vi "Process_DoNotRun.vi"(8 "error in":errorcluster, 11 "Logger":refnum<class "Logger.lvclass">) -> (0 "error out":errorcluster, 3 "Logger out":refnum<class "Logger.lvclass">)   [LabVIEW 2019, in "Logger.lvclass"]
doc: "---------------------------------------------------------------\nJKI State Machine Objects™\nhttp://jki.net/state-machine-objects/\nCopyright (C) 2005-2015, JKI <info@jki.net>\nALL RIGHTS RESERVED"
uses:
  Logger.lvclass
  <vilib>/JKI/JKI SMO/SMO/SMO.lvclass
  C:/Program Files (x86)/National Instruments/LabVIEW 2019/vi.lib/JKI/JKI SMO/SMO/SMO.lvclass
panel:
  out "String":string
  # "For instructions on how to use the JKI State Machine Objects, examples and video tutorials, visit:\nhttp://jki.net/state-machine-objects/\n\nJKI State Machine Objects™\nhttp://jki.net/state-machine-objects/\nCopyright (C) 2005-2015, JKI <info@jki.net>\nALL RIGHTS RESERVED"
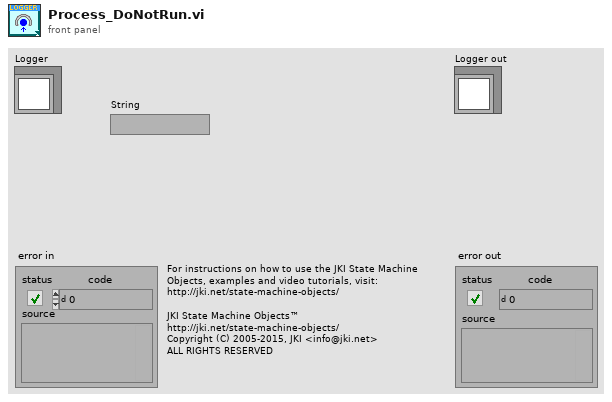
[diagram p1: front panel]
types:
  T1 = enum32{"invalid app kind", "Development System", "Run Time System", "Student Edition", "Embedded LabVIEW", "Evaluation", "Custom"}
  T2 = enum32{"Invalid", "Standard", "Closed", "Hidden", "Minimized", "Maximized"}
  T3 = enum32{"Bad", "Idle", "Run top level", "Running"}
  T4 = cluster{"Core":cluster{"Current VI Reference":refnum<vi>, "Close Panel on Exit?":bool, "error":errorcluster}, "Self Reference":refnum<class "Logger.lvclass">, "Debug Mode?":bool}
  T5 = cluster{"Current VI Reference":refnum<vi>, "Close Panel on Exit?":bool, "error":errorcluster}
  T6 = typedef "SMO.lvclass/Protected Events.ctl" = cluster{"StopProcesses":refnum<user-event>, "AbortProcesses":refnum<user-event>, "Config Changed":refnum<user-event>, "Dependency":refnum<user-event>}
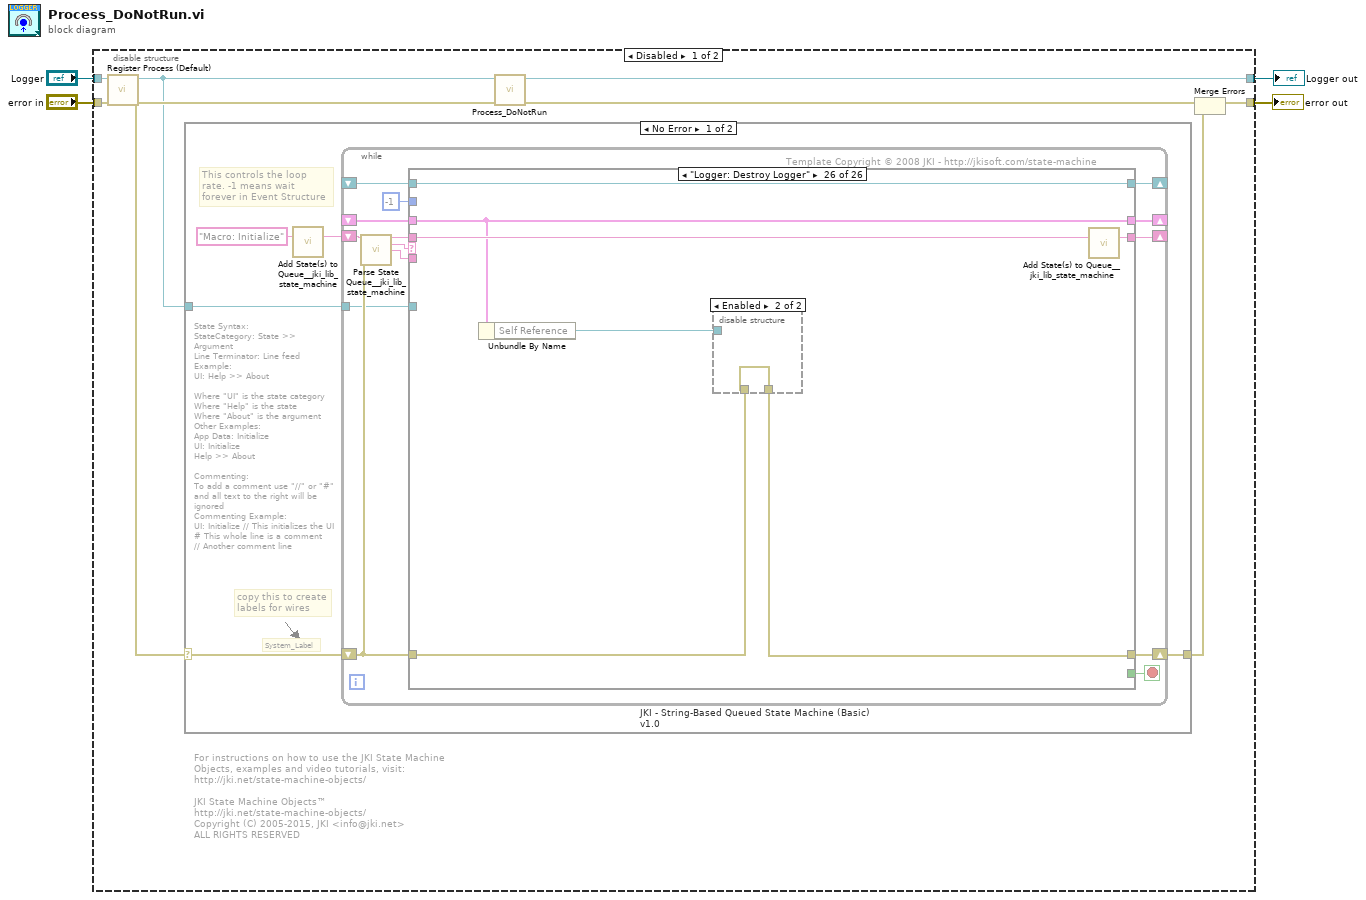
[diagram p0: block diagram]
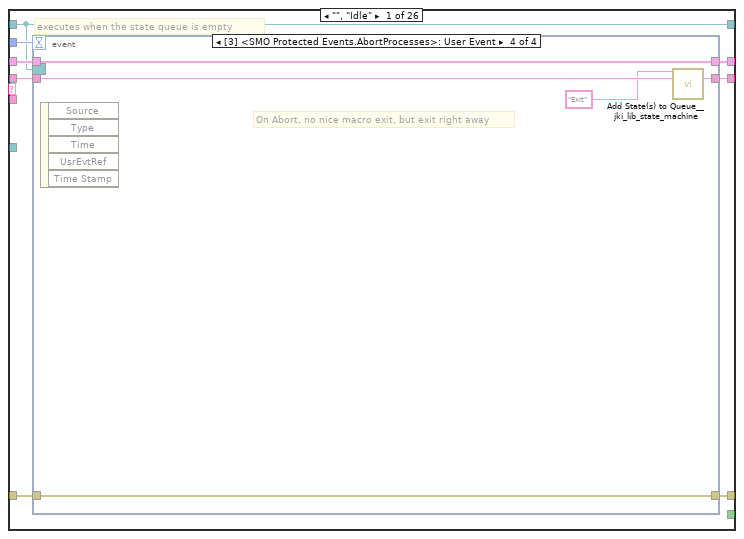
[diagram p2: hidden frame]
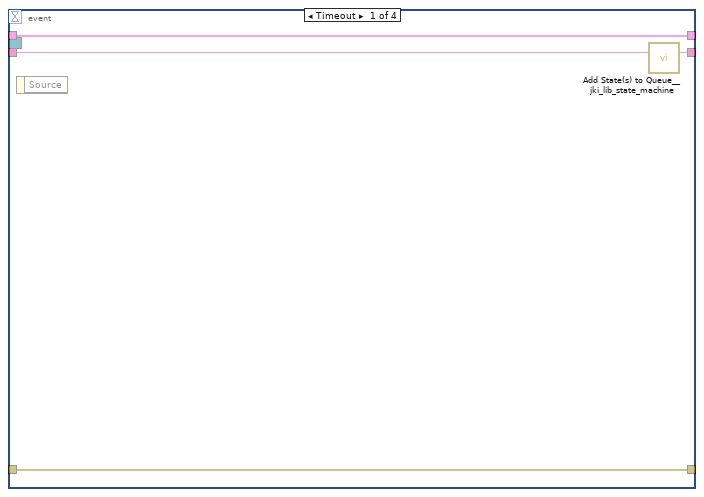
[diagram p3: hidden frame]
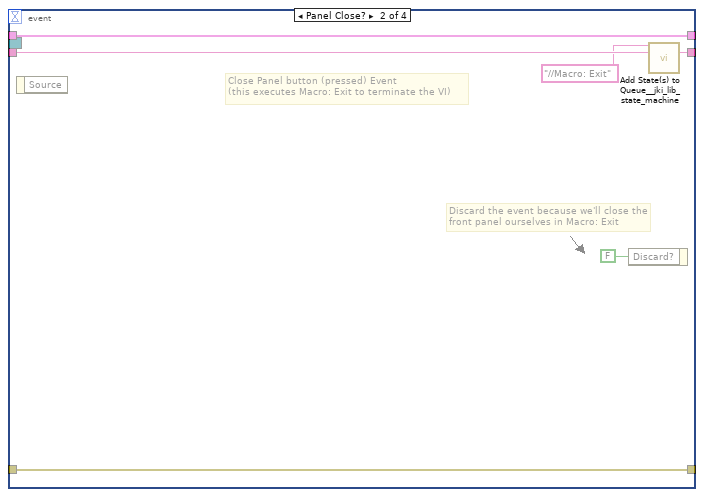
[diagram p4: hidden frame]
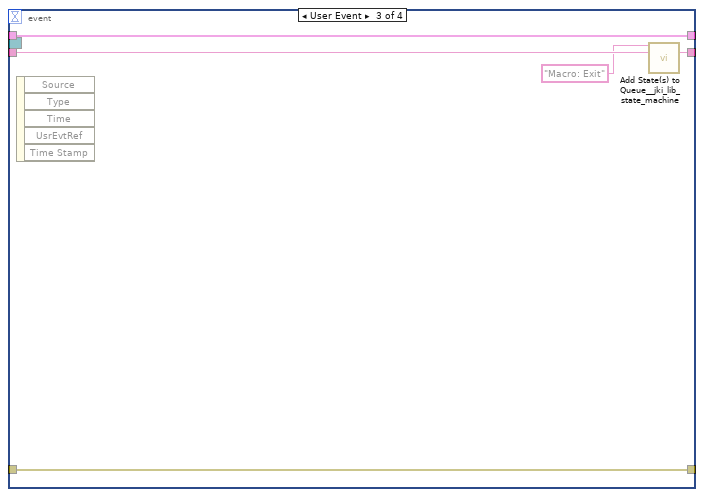
[diagram p5: hidden frame]
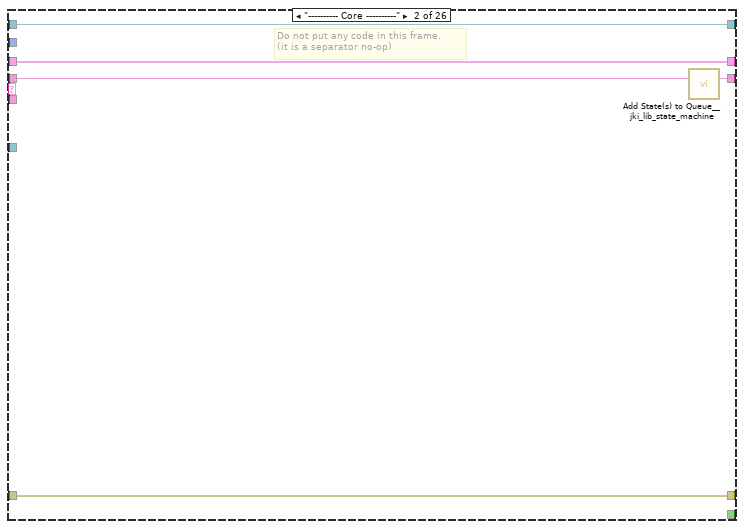
[diagram p6: hidden frame]
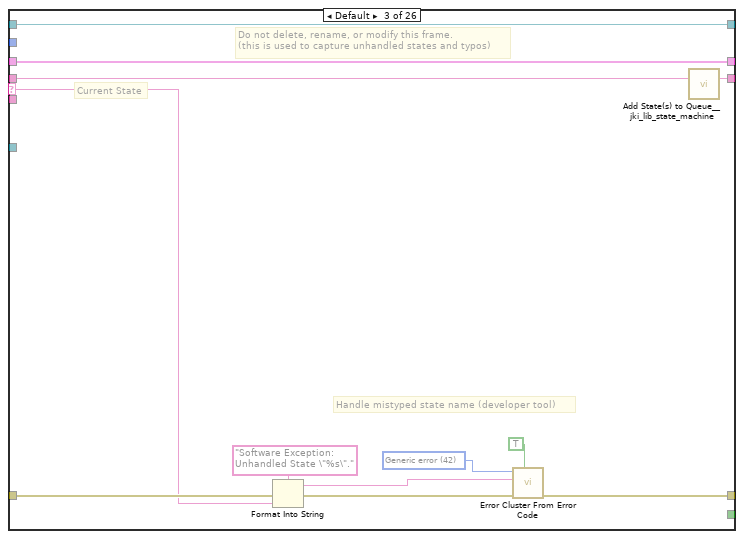
[diagram p7: hidden frame]
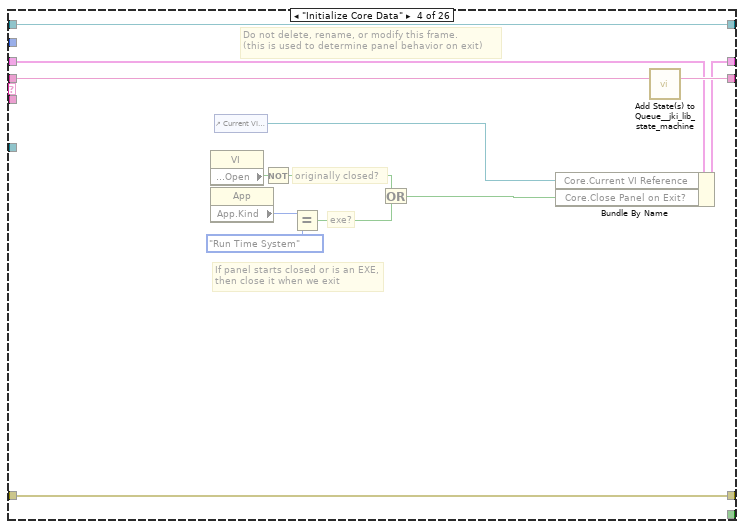
[diagram p8: hidden frame]
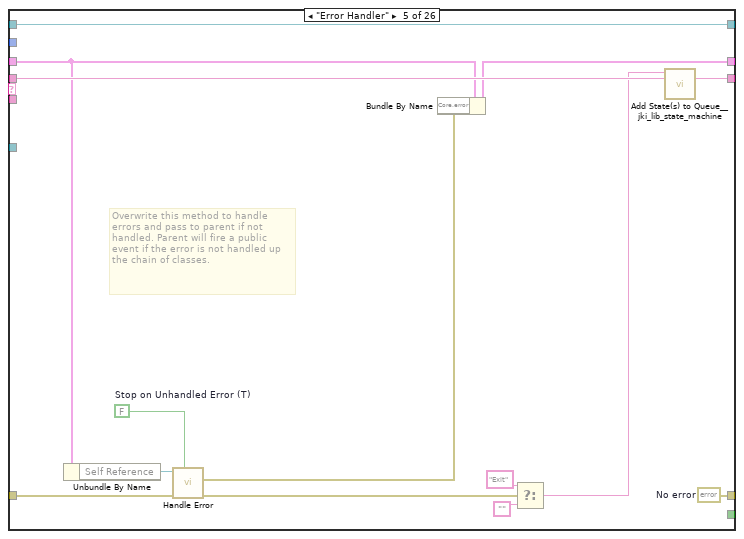
[diagram p9: hidden frame]
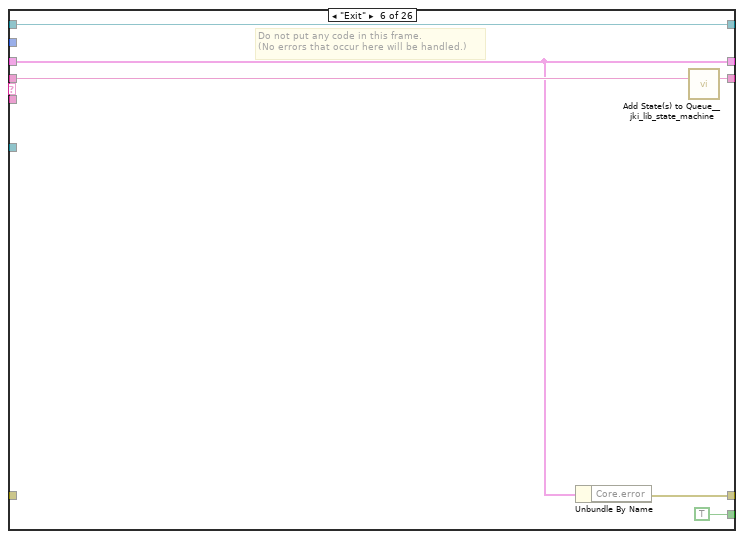
[diagram p10: hidden frame]
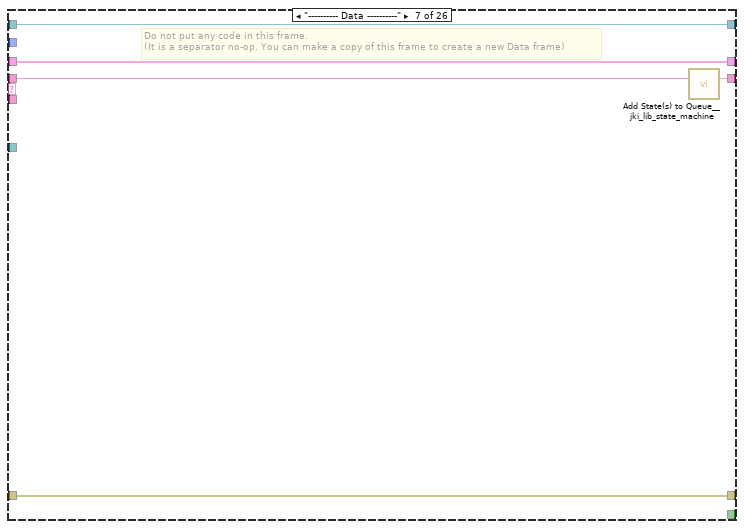
[diagram p11: hidden frame]
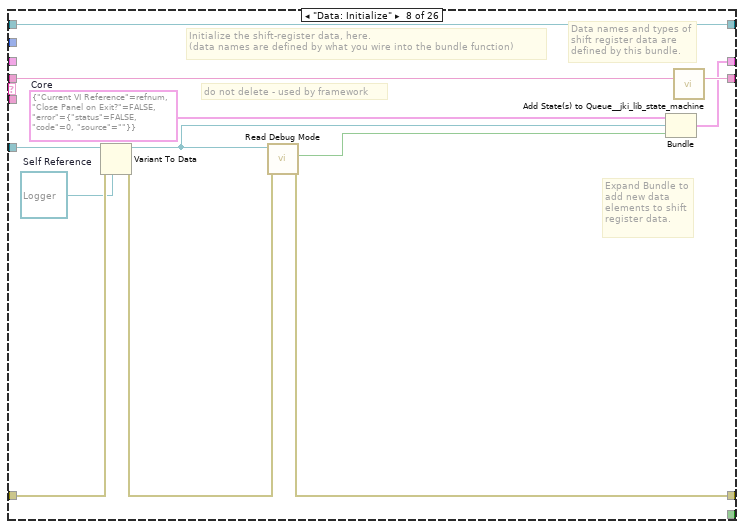
[diagram p12: hidden frame]
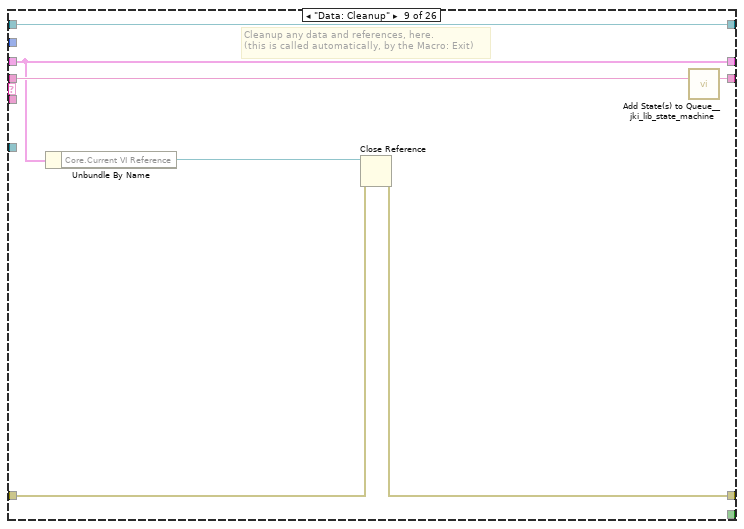
[diagram p13: hidden frame]
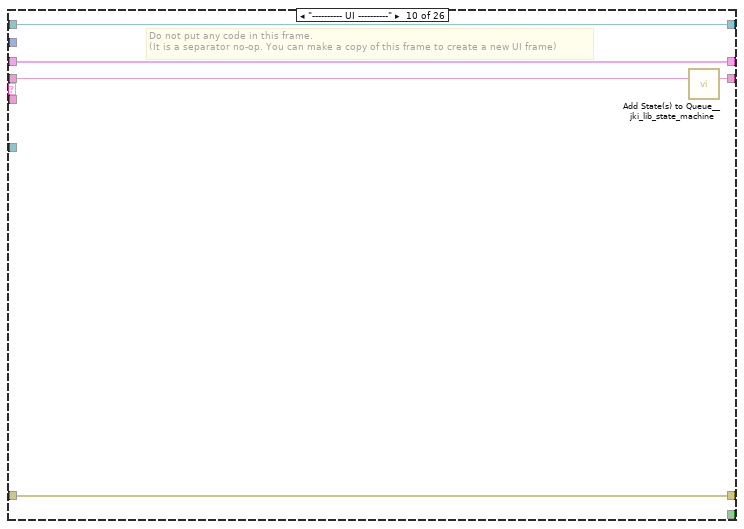
[diagram p14: hidden frame]
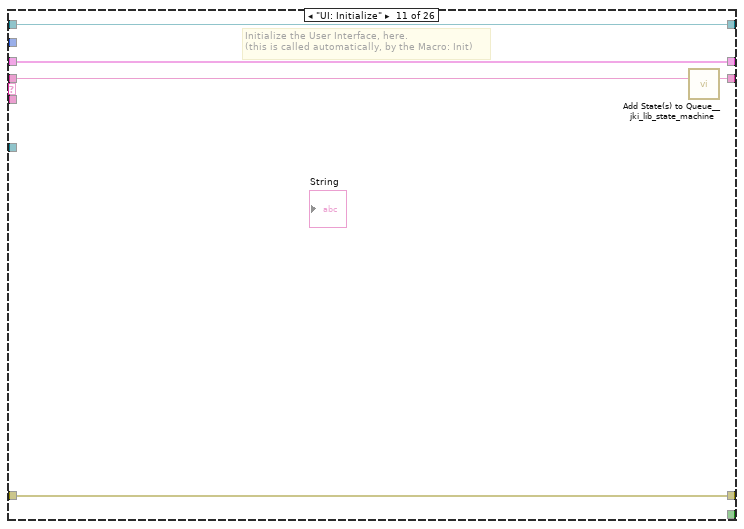
[diagram p15: hidden frame]
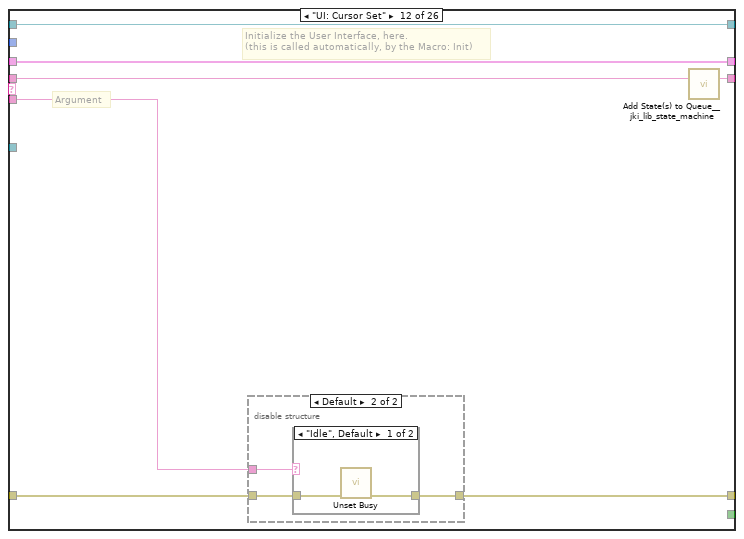
[diagram p16: hidden frame]
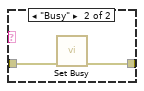
[diagram p18: hidden frame]
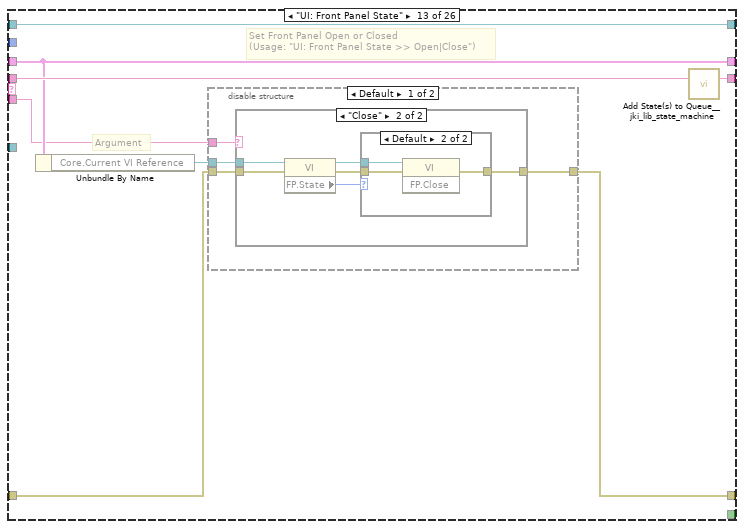
[diagram p19: hidden frame]
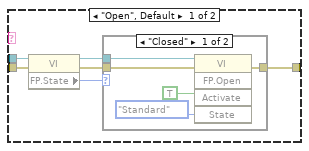
[diagram p20: hidden frame]
diagram:
  n1 = disable-structure shown="Disabled" {
    disable-tunnel: "Logger" -> [w12 w321]
    disable-tunnel: "error in" -> [w11 w320]
    disable-tunnel: [w10 w320] -> w2
    disable-tunnel: [w7 w321] -> w1
    frame Disabled {
      # "For instructions on how to use the JKI State Machine Objects, examples and video tutorials, visit:\nhttp://jki.net/state-machine-objects/\n\nJKI State Machine Objects™\nhttp://jki.net/state-machine-objects/\nCopyright (C) 2005-2015, JKI <info@jki.net>\nALL RIGHTS RESERVED"
      n2 = call <vilib>:"Register Process (Default).vi"("error in (no error)"=w11, "SMO"=w12) -> ("error out"=w9:errorcluster, "SelfRef"=w8:refnum<class "Logger.lvclass">)  [unwired: 8 in]
      n3 = case shown="No Error" w9 {
        selector: w9 -> [w14 w319]
        tunnel: w8 -> [w15 _]
        tunnel: [w13 w319] -> w5
        frame No Error {
          # "State Syntax:\nStateCategory: State >> Argument\nLine Terminator: Line feed\nExample:\nUI: Help >> About\n\nWhere \"UI\" is the state category\nWhere \"Help\" is the state\nWhere \"About\" is the argument\nOther Examples:\nApp Data: Initialize\nUI: Initialize\nHelp >> About\n\nCommenting:\nTo add a comment use \"//\" or \"#\" and all text to the right will be ignored\nCommenting Example:\nUI: Initialize // This initializes the UI\n# This whole line is a comment\n// Another comment line"
          # "copy this to create labels for wires"
          # "This controls the loop rate. -1 means wait forever in Event Structure"
          # "System_Label"
          n4 = call <vilib>:"Add State(s) to Queue__jki_lib_state_machine.vi"("State(s) in (\"\")"="Macro: Initialize") -> ("States Out"=w17:string)  [unwired: 14 in]
          n5 = while "JKI - String-Based Queued State Machine (Basic) v1.0" {
            shift-right: [w24] -> _
            shift-left: _ -> [w23]
            shift-right: [w27] -> w13
            shift-left: w14 -> [w21]
            shift-right: [w26] -> _
            shift-left: w17 -> [w28]
            tunnel: w15 -> [w20]
            shift-right: [w19] -> _
            shift-left: _ -> [w18]
            stop <- w25 stop-if-true
            # "Template Copyright © 2008 JKI - http://jkisoft.com/state-machine"
            n6 = call <vilib>:"Parse State Queue__jki_lib_state_machine.vi"("State Queue"=w28, "Error In (no error)"=w21) -> ("Remaining States"=w30:string, "Current State"=w31:string, "Arguments"=w29:string)  [unwired: 11 in]
            n7 = case shown="\"Logger: Destroy Logger\"" w31 {
              selector: w31 -> [_ _ w66 _ _ _ _ _ _ _ _ _ _ _ _ _ _ _ _ _ _ _ _ _ _ _]
              tunnel: w30 -> [w39 w64 w70 w89 w103 w109 w114 w126 w133 w138 w143 w150 w166 w198 w221 w240 w245 w256 w261 w271 w277 w282 w291 w302 w307 w314]
              tunnel: w29 -> [_ _ _ _ _ _ _ _ _ _ _ w144 w160 _ _ _ _ _ _ _ _ _ _ _ _ _]
              tunnel: w23 -> [w37 w61 w68 w80 w97 w105 w111 _ w128 w135 w141 w148 w162 w195 w203 w232 w242 w246 w258 w269 w275 w280 w288 w298 w303 w311]
              tunnel: [w36 w62 w72 w86 w98 w104 w112 w115 w129 w136 w140 w145 w163 w196 w199 w238 w243 w248 w259 w264 w273 w278 w283 w299 w304 w308] -> w27
              tunnel: w21 -> [w35 w62 w71 w86 w99 _ w112 w123 w130 w136 w140 w146 w164 w196 w200 w238 w243 w249 w259 w265 w273 w278 w284 w299 w304 w309]
              tunnel: [w38 w63 w69 w88 w102 w108 w113 w125 w132 w137 w142 w149 w165 w197 w220 w239 w244 w255 w260 w270 w276 w281 w290 w301 w306 w313] -> w26
              tunnel: [_ _ _ _ _ TRUE _ _ _ _ _ _ _ _ _ _ _ _ _ _ _ _ _ _ _ _] -> w25
              tunnel: [w34 w61 w68 w87 w96 w105 w111 w124 w128 w135 w141 w148 w162 w195 w203 w232 w242 w246 w258 w269 w275 w280 w287 w298 w303 w311] -> w24
              tunnel: -1 ("Timeout") -> [w33 _ _ _ _ _ _ _ _ _ _ _ _ _ _ _ _ _ _ _ _ _ _ _ _ _]
              tunnel: w20 -> [_ _ _ _ _ _ _ w121 _ _ _ _ _ _ w201 _ _ _ _ _ _ _ _ _ _ _]
              tunnel: [w32 w60 w65 w77 w101 w106 w110 w120 w127 w134 w139 w147 w159 w194 w219 w233 w241 w254 w257 w268 w274 w279 w289 w300 w305 w312] -> w19
              tunnel: w18 -> [w32 w60 w65 w77 w101 w106 w110 w120 w127 w134 w139 w147 w159 w194 w219 w233 w241 w254 w257 _ w274 w279 w289 w300 w305 w312]
              frame "", "Idle" {
                # "executes when the state queue is empty"
                n8 = event shown="[3] <SMO Protected Events.AbortProcesses>: User Event" {
                  selector: w32 -> [_ _ _ _]
                  dyn-events: _ -> [_ _ _ _]
                  timeout: w33 -> [_ _ _ _]
                  tunnel: w39 -> [w43 w49 w54 w59]
                  tunnel: [w42 w48 w53 w58] -> w38
                  tunnel: w37 -> [w41 w46 w51 w56]
                  tunnel: [w40 w47 w52 w57] -> w36
                  tunnel: w35 -> [w40 w47 w52 w57]
                  tunnel: [w41 w46 w51 w56] -> w34
                  event Timeout {
                    n9 = event-data() -> ()  [unwired: 1 in, 1 out]
                    n10 = call <vilib>:"Add State(s) to Queue__jki_lib_state_machine.vi"("State(s) in (\"\")"=w43) -> ("States Out"=w42:string)  [unwired: 14 in]
                  }
                  event Panel Close? {
                    # "Discard the event because we'll close the front panel ourselves in Macro: Exit"
                    # "Close Panel button (pressed) Event\n(this executes Macro: Exit to terminate the VI)"
                    n11 = event-data() -> ()  [unwired: 1 in, 1 out]
                    n12 = event-data("Discard?"=FALSE) -> ()  [unwired: 1 in, 1 out]
                    n13 = call <vilib>:"Add State(s) to Queue__jki_lib_state_machine.vi"("State(s) in Front (\"\")"="//Macro: Exit", "State(s) in (\"\")"=w49) -> ("States Out"=w48:string)  [unwired: 13 in]
                  }
                  event User Event {
                    n14 = event-data() -> ()  [unwired: 1 in, 5 out]
                    n15 = call <vilib>:"Add State(s) to Queue__jki_lib_state_machine.vi"("State(s) in Front (\"\")"="Macro: Exit", "State(s) in (\"\")"=w54) -> ("States Out"=w53:string)  [unwired: 13 in]
                  }
                  event User Event {
                    # "On Abort, no nice macro exit, but exit right away"
                    n16 = event-data() -> ()  [unwired: 1 in, 5 out]
                    n17 = call <vilib>:"Add State(s) to Queue__jki_lib_state_machine.vi"("State(s) in Front (\"\")"="Exit", "State(s) in (\"\")"=w59) -> ("States Out"=w58:string)  [unwired: 13 in]
                  }
                }
              }
              frame "---------- Core ----------" {
                # "Do not put any code in this frame.\n(it is a separator no-op)"
                n18 = call <vilib>:"Add State(s) to Queue__jki_lib_state_machine.vi"("State(s) in (\"\")"=w64) -> ("States Out"=w63:string)  [unwired: 14 in]
              }
              frame Default {
                w75 = 42 items=["No error", "Argument error", "Memory is full", "Out of zone", "End of file", "File already open", "Generic file I/O error", "File not found", "File permission error", "Disk is full", "Duplicate path", "Too many files open", "System feature not enabled", "Resource file not found", "Cannot add resource", "Resource not found", "Image not found", "Image memory error", "Pen does not exist", "Config type invalid", "Config token not found", "Config parse error", "Config memory error", "Bad external code format", "Bad external code offset", "External code not present", "Null window", "Destroy window error", "Null menu", "Print aborted", "Bad print record", "Print driver error", "Windows error during printing", "Memory error during printing", "Print dialog error", "Generic print error", "Invalid device refnum", "Device not found", "Device parameter error", "Device unit error", "Cannot open device", "Device call aborted", "Generic error", "Cancelled by user", "Object ID too low", "Object ID too high", "Object not in heap", "Unknown heap", "Unknown object (invalid DefProc)", "Unknown object (DefProc not in table)", "Message out of range", "Invalid (null) method", "Unknown message", "Manager call not supported", "Bad address", "Network operation in progress", "Network operation timed out", "Connection is busy", "Network attribute not supported", "Network error", "Address in use", "System out of memory", "Connection aborted", "Connection refused", "Not connected", "Already connected", "Connection closed", "Initialization error (interapplication manager)", "Bad occurrence", "Wait on unbound occurrence handler", "Occurrence queue overflow", "Datalog type conflict", "Unused", "Unrecognized type (interapplication manager)", "Memory corrupt", "Failed to make temporary DLL", "Old CIN version", "Drag socket not found", "Failed to load drop-object", "Failed to register OLE object", "Failed to release OLE object", "Format specifier type mismatch", "Unknown format specifier", "Too few format specifiers", "Too many format specifiers", "Scan failed", "Newer CIN version", "Error converting to variant", "Runtime menu error", "Password tampered", "Variant attribute not found", "Incompatible variant data type", "Event data is not available", "Event Store is not present", "Occurrence is not found", "Event Queue is not created", "Event info is not available", "Refnum passed is NULL", "Error retrieving Class GUID", "Error retrieving CoClass GUID", "Error retrieving TypeLib GUID.", "Bad built application magic bytes.", "Specific driver is different from the specific driver associated with the Logical Name.", "There is no session opened to the class driver.", "Max Error", "MAX - Error with config objects", "MAX - Error loading configuration", "MAX - Group not supported"]
                # "Current State"
                # "Do not delete, rename, or modify this frame.\n(this is used to capture unhandled states and typos)"
                # "Handle mistyped state name (developer tool)"
                n19 = Format Into String(format string="Software Exception: Unhandled State \"%s\"." ("message"), error in=w71, w66) -> (resulting string=w74:string, error out=w73:errorcluster)  [unwired: 1 in]
                n20 = call <vilib>:"Error Cluster From Error Code.vi"("show call chain? (False)"=TRUE, "error in (no error)"=w73, "error message (\"\")"=w74, "error code (0)"=w75) -> ("error out"=w72:errorcluster)  [unwired: 5 in]
                n21 = call <vilib>:"Add State(s) to Queue__jki_lib_state_machine.vi"("State(s) in (\"\")"=w70) -> ("States Out"=w69:string)  [unwired: 14 in]
              }
              frame "Initialize Core Data" {
                # "Do not delete, rename, or modify this frame.\n(this is used to determine panel behavior on exit)"
                # "originally closed?"
                # "exe?"
                # "If panel starts closed or is an EXE, then close it when we exit"
                n22 = property class="VI"() -> ("Front Panel.Open"=w85:bool)  [unwired: 2 in, 2 out]
                n23 = property class="App"() -> ("App.Kind"=w84:T1)  [unwired: 2 in, 2 out]
                n24 = control-ref of="Current VI Reference"() -> (w78:refnum<vi>)
                n25 = Not(x=w85) -> (.not. x?=w82:bool)
                n26 = Equal?(x=w84, y=T1."Run Time System" ("Application:Kind")) -> (x = y?=w81:bool)
                n27 = Or(x=w82, y=w81) -> (x .or. y?=w79:bool)
                n28 = Bundle By Name(cluster=w80, "Core.Current VI Reference"=w78, "Core.Close Panel on Exit?"=w79) -> (w87:T4)
                n29 = call <vilib>:"Add State(s) to Queue__jki_lib_state_machine.vi"("State(s) in (\"\")"=w89) -> ("States Out"=w88:string)  [unwired: 14 in]
              }
              frame "Error Handler" {
                w90 = FALSE  # Stop on Unhandled Error (T)
                w98 = errorcluster {"status"=FALSE, "code"=0, "source"=""}  # No error
                # "Overwrite this method to handle errors and pass to parent if not handled. Parent will fire a public event if the error is not handled up the chain of classes."
                n30 = Unbundle By Name(w97) -> ("Self Reference"=w100:refnum<class "Logger.lvclass">)
                n31 = call-dynamic "Handle Error.vi"("Stop on Unhandled Error (T)"=w90, "error in"=w99, "SMO"=w100) -> ("handling error"=w91:errorcluster, "Unhandled error"=w94:errorcluster)  [unwired: 6 in, 1 out]
                n32 = Bundle By Name(cluster=w97, "Core.error"=w94) -> (w96:T4)
                n33 = Select(t="Exit", s=w91, f="") -> (s? t:f=w95:string)
                n34 = call <vilib>:"Add State(s) to Queue__jki_lib_state_machine.vi"("State(s) in Front (\"\")"=w95, "State(s) in (\"\")"=w103) -> ("States Out"=w102:string)  [unwired: 13 in]
              }
              frame "Exit" {
                # "Do not put any code in this frame.\n(No errors that occur here will be handled.)"
                n35 = Unbundle By Name(w105) -> ("Core.error"=w104:errorcluster)
                n36 = call <vilib>:"Add State(s) to Queue__jki_lib_state_machine.vi"("State(s) in (\"\")"=w109) -> ("States Out"=w108:string)  [unwired: 14 in]
              }
              frame "---------- Data ----------" {
                # "Do not put any code in this frame.\n(It is a separator no-op. You can make a copy of this frame to create a new Data frame)"
                n37 = call <vilib>:"Add State(s) to Queue__jki_lib_state_machine.vi"("State(s) in (\"\")"=w114) -> ("States Out"=w113:string)  [unwired: 14 in]
              }
              frame "Data: Initialize" {
                w119 = T5 {"Current VI Reference"=refnum, "Close Panel on Exit?"=FALSE, "error"={"status"=FALSE, "code"=0, "source"=""}}  # Core
                w122 = refnum<class "Logger.lvclass"> refnum  # Self Reference
                # "do not delete - used by framework"
                # "Expand Bundle to add new data elements to shift register data."
                # "Data names and types of shift register data are defined by this bundle."
                # "Initialize the shift-register data, here.\n(data names are defined by what you wire into the bundle function)"
                n38 = Variant To Data(error in=w123, type=w122, Variant=w121) -> (data=w118:refnum<class "Logger.lvclass">, error out=w116:errorcluster)
                n39 = call "Read Debug Mode.vi"("error in (no error)"=w116, "Logger in"=w118) -> ("error out"=w115:errorcluster, "Debug Mode?"=w117:bool)  [unwired: 7 in, 1 out]
                n40 = Bundle("Core"=w119, "Self Reference"=w118, "Debug Mode?"=w117) -> (w124:T4)  [unwired: 1 in]
                n41 = call <vilib>:"Add State(s) to Queue__jki_lib_state_machine.vi"("State(s) in (\"\")"=w126) -> ("States Out"=w125:string)  [unwired: 14 in]
              }
              frame "Data: Cleanup" {
                # "Cleanup any data and references, here.\n(this is called automatically, by the Macro: Exit)"
                n42 = Unbundle By Name(w128) -> ("Core.Current VI Reference"=w131:refnum<vi>)
                n43 = Close Reference(reference=w131, error in (no error)=w130) -> (error out=w129:errorcluster)
                n44 = call <vilib>:"Add State(s) to Queue__jki_lib_state_machine.vi"("State(s) in (\"\")"=w133) -> ("States Out"=w132:string)  [unwired: 14 in]
              }
              frame "---------- UI ----------" {
                # "Do not put any code in this frame.\n(It is a separator no-op. You can make a copy of this frame to create a new UI frame)"
                n45 = call <vilib>:"Add State(s) to Queue__jki_lib_state_machine.vi"("State(s) in (\"\")"=w138) -> ("States Out"=w137:string)  [unwired: 14 in]
              }
              frame "UI: Initialize" {
                # "Initialize the User Interface, here.\n(this is called automatically, by the Macro: Init)"
                n46 = call <vilib>:"Add State(s) to Queue__jki_lib_state_machine.vi"("State(s) in (\"\")"=w143) -> ("States Out"=w142:string)  [unwired: 14 in]
              }
              frame "UI: Cursor Set" {
                # "Argument"
                # "Initialize the User Interface, here.\n(this is called automatically, by the Macro: Init)"
                n47 = disable-structure shown="Default" {
                  disable-tunnel: w146 -> [w151 w154]
                  disable-tunnel: [w151 w153] -> w145
                  disable-tunnel: w144 -> [_ w152]
                  frame condition #0 {
                  }
                  frame condition #1 (active) {
                    n48 = case shown="\"Idle\", Default" w152 {
                      tunnel: w154 -> [w156 w158]
                      tunnel: [w155 w157] -> w153
                      frame "Idle", Default {
                        n49 = call <vilib>:"Unset Busy.vi"("error in (no error)"=w156) -> ("error out"=w155:errorcluster)  [unwired: 10 in]
                      }
                      frame "Busy" {
                        n50 = call <vilib>:"Set Busy.vi"("error in (no error)"=w158) -> ("error out"=w157:errorcluster)  [unwired: 9 in, 1 out]
                      }
                    }
                  }
                }
                n51 = call <vilib>:"Add State(s) to Queue__jki_lib_state_machine.vi"("State(s) in (\"\")"=w150) -> ("States Out"=w149:string)  [unwired: 14 in]
              }
              frame "UI: Front Panel State" {
                # "Argument"
                # "Set Front Panel Open or Closed\n(Usage: \"UI: Front Panel State >> Open|Close\")"
                n52 = Unbundle By Name(w162) -> ("Core.Current VI Reference"=w161:refnum<vi>)
                n53 = disable-structure shown="Default" {
                  disable-tunnel: w164 -> [w170 w193]
                  disable-tunnel: [w169 w193] -> w163
                  disable-tunnel: w161 -> [w168 _]
                  disable-tunnel: w160 -> [w167 _]
                  frame condition #0 (active) {
                    n54 = case shown="\"Close\"" w167 {
                      tunnel: w170 -> [w174 w187]
                      tunnel: [w176 w188] -> w169
                      tunnel: w168 -> [w175 w185]
                      frame "Open", Default {
                        n55 = property class="VI"(reference=w175, error in=w174) -> (reference out=w172:refnum<vi>, error out=w173:errorcluster, "FP.State"=w171:T2)
                        n56 = case shown="\"Closed\"" w171 {
                          tunnel: [w179 w182] -> w176
                          tunnel: w173 -> [w178 w182]
                          tunnel: w172 -> [w177 _]
                          frame "Closed" {
                            n57 = invoke class="VI" method="FP.Open"(reference=w177, error in=w178, "Activate"=TRUE, "State"=T2."Standard") -> (error out=w179:errorcluster)  [unwired: 1 in, 4 out]
                          }
                          frame Default {
                          }
                        }
                      }
                      frame "Close" {
                        n58 = property class="VI"(reference=w185, error in=w187) -> (reference out=w184:refnum<vi>, error out=w186:errorcluster, "FP.State"=w183:T2)
                        n59 = case shown="Default" w183 {
                          tunnel: [w189 w192] -> w188
                          tunnel: w186 -> [w189 w191]
                          tunnel: w184 -> [_ w190]
                          frame "Invalid", "Closed" {
                          }
                          frame Default {
                            n60 = invoke class="VI" method="FP.Close"(reference=w190, error in=w191) -> (error out=w192:errorcluster)  [unwired: 1 in, 2 out]
                          }
                        }
                      }
                    }
                  }
                  frame condition #1 {
                  }
                }
                n61 = call <vilib>:"Add State(s) to Queue__jki_lib_state_machine.vi"("State(s) in (\"\")"=w166) -> ("States Out"=w165:string)  [unwired: 14 in]
              }
              frame "---------- Macro ----------" {
                # "Do not put any code in this frame.\n(It is a separator no-op. You can make a copy of this frame to create a new Macro frame)"
                n62 = call <vilib>:"Add State(s) to Queue__jki_lib_state_machine.vi"("State(s) in (\"\")"=w198) -> ("States Out"=w197:string)  [unwired: 14 in]
              }
              frame "Macro: Initialize" {
                w211 = "Process: Sync"
                # "This needs to be called here before Data: Initialize\nto ensure that the correct argument is present"
                # "Initialization Macro\n(This is called once, when the VI starts)"
                n63 = control-ref of="This VI"() -> (w213:refnum<vi>)
                n64 = property class="VI"(reference=w213) -> ("Exec.State"=w212:T3)  [unwired: 1 in, 2 out]
                n65 = call "Read Debug Mode.vi"("error in (no error)"=w200, "Logger in"=w201) -> ("error out"=w199:errorcluster, "Debug Mode?"=w202:bool)  [unwired: 7 in, 1 out]
                n66 = Equal?(x=w212, y=T3."Run top level") -> (x = y?=w217:bool)
                n67 = Select(t="Open", s=w202, f="Close") -> (s? t:f=w208:string)
                n68 = call <vilib>:"Build State String with Arguments__JKI_lib_State_Machine.vi"("Arguments (\"\")"=w208, "State"="UI: Front Panel State") -> ("State with Arguments"=w206:string)  [unwired: 4 in]
                n69 = Select(t=w211, s=w217, f="") -> ()  [unwired: 1 out]
                n70 = call <vilib>:"Add State(s) to Queue__jki_lib_state_machine.vi"("State(s) in Front (\"\")"="Logger: Create Logger\nUI: Initialize", "State(s) in (\"\")"=w206) -> ("States Out"=w204:string)  [unwired: 13 in]
                n71 = call <vilib>:"Add State(s) to Queue__jki_lib_state_machine.vi"("State(s) in Front (\"\")"="Data: Initialize\nInitialize Core Data\nEvents: Register", "State(s) in (\"\")"=w211, "State(s) at Back (\"\")"=w204) -> ("States Out"=w214:string)  [unwired: 12 in]
                n72 = call <vilib>:"Add State(s) to Queue__jki_lib_state_machine.vi"("State(s) in Front (\"\")"=w214, "State(s) in (\"\")"=w221) -> ("States Out"=w220:string)  [unwired: 13 in]
              }
              frame "Macro: Exit" {
                # "Exit Macro\n(This is called once, when the VI exits)"
                n73 = Unbundle By Name(w232) -> ("Debug Mode?"=w222:bool, "Core.Close Panel on Exit?"=w237:bool)
                n74 = Select(t="Open", s=w222, f="Close") -> (s? t:f=w225:string)
                n75 = call <vilib>:"Build State String with Arguments__JKI_lib_State_Machine.vi"("Arguments (\"\")"=w225, "State"="UI: Front Panel State") -> ("State with Arguments"=w223:string)  [unwired: 4 in]
                n76 = Select(t=w223, s=w237, f="") -> (s? t:f=w235:string)
                n77 = call <vilib>:"Add State(s) to Queue__jki_lib_state_machine.vi"("State(s) in Front (\"\")"="Logger: Destroy Logger\nData: Cleanup\nEvents: Unregister", "State(s) in (\"\")"="Process: Sync", "State(s) at Back (\"\")"="Exit") -> ("States Out"=w229:string)  [unwired: 12 in]
                n78 = call <vilib>:"Add State(s) to Queue__jki_lib_state_machine.vi"("State(s) in (\"\")"=w235, "State(s) at Back (\"\")"=w229) -> ("States Out"=w234:string)  [unwired: 13 in]
                n79 = call <vilib>:"Add State(s) to Queue__jki_lib_state_machine.vi"("State(s) in Front (\"\")"=w234, "State(s) in (\"\")"=w240) -> ("States Out"=w239:string)  [unwired: 13 in]
              }
              frame "---------- Process ----------" {
                # "Template Separator\n(You can make a copy of, or modify, this frame)"
                n80 = call <vilib>:"Add State(s) to Queue__jki_lib_state_machine.vi"("State(s) in (\"\")"=w245) -> ("States Out"=w244:string)  [unwired: 14 in]
              }
              frame "Process: Sync" {
                n81 = Unbundle By Name(w246) -> ("Self Reference"=w250:refnum<class "Logger.lvclass">)
                n82 = call <vilib>:"WaitOnProcessSync.vi"("error in (no error)"=w249, "SMO"=w250) -> ("error out"=w248:errorcluster, "Don't run?"=w253:bool)  [unwired: 7 in, 1 out]
                n83 = Select(t="Data: Cleanup\nEvents: Unregister\nExit", s=w253, f="") -> (s? t:f=w247:string)
                n84 = call <vilib>:"Add State(s) to Queue__jki_lib_state_machine.vi"("State(s) in Front (\"\")"=w247, "State(s) in (\"\")"=w256) -> ("States Out"=w255:string)  [unwired: 13 in]
              }
              frame "---------- Events ----------" {
                # "Template Separator\n(You can make a copy of, or modify, this frame)"
                n85 = call <vilib>:"Add State(s) to Queue__jki_lib_state_machine.vi"("State(s) in (\"\")"=w261) -> ("States Out"=w260:string)  [unwired: 14 in]
              }
              frame "Events: Register" {
                # "Expand to add\nmore events"
                n86 = Unbundle By Name(w269) -> ("Self Reference"=w266:refnum<class "Logger.lvclass">)
                n87 = call <vilib>:"GetProtectedEvents.vi"("SMO"=w266) -> ("error out"=w262:errorcluster, "SMO Protected Events"=w267:T6)  [unwired: 8 in, 1 out]
                n88 = register-events(w267) -> (reference out=w268:refnum<event-registration>, error out=w263:errorcluster)  [unwired: 2 in]
                n89 = Merge Errors(w265, w263, w262) -> (w264:errorcluster)
                n90 = call <vilib>:"Add State(s) to Queue__jki_lib_state_machine.vi"("State(s) in (\"\")"=w271) -> ("States Out"=w270:string)  [unwired: 14 in]
              }
              frame "Events: Unregister" {
                n91 = Unregister For Events(event registration refnum=w274, error in=w273) -> (error out=w272:errorcluster)
                n92 = call <vilib>:"Clear Errors.vi"("error in (no error)"=w272) -> ()  [unwired: 5 in, 2 out]
                n93 = call <vilib>:"Add State(s) to Queue__jki_lib_state_machine.vi"("State(s) in (\"\")"=w277) -> ("States Out"=w276:string)  [unwired: 14 in]
              }
              frame "---------- Logger ----------" {
                n94 = call <vilib>:"Add State(s) to Queue__jki_lib_state_machine.vi"("State(s) in (\"\")"=w282) -> ("States Out"=w281:string)  [unwired: 14 in]
              }
              frame "Logger: Create Logger" {
                n95 = Unbundle By Name(w288) -> ("Self Reference"=w286:refnum<class "Logger.lvclass">)
                n96 = disable-structure shown="Enabled" {
                  disable-tunnel: w286 -> [w295 w297]
                  disable-tunnel: [w294 w297] -> w285
                  disable-tunnel: w284 -> [w293 w296]
                  disable-tunnel: [w292 w296] -> w283
                  frame Disabled {
                    n97 = call-dynamic "Create Logger.vi"("error in (no error)"=w293, "Logger in"=w295) -> ("error out"=w292:errorcluster, "Logger out"=w294:refnum<class "Logger.lvclass">)  [unwired: 8 in]
                  }
                  frame Enabled {
                  }
                }
                n98 = Bundle By Name(cluster=w288, "Self Reference"=w285) -> (w287:T4)
                n99 = call <vilib>:"Add State(s) to Queue__jki_lib_state_machine.vi"("State(s) in (\"\")"=w291) -> ("States Out"=w290:string)  [unwired: 14 in]
              }
              frame "Logger: Write Logger" {
                n100 = Unbundle By Name(w298) -> ()  [unwired: 1 out]
                n101 = call <vilib>:"Add State(s) to Queue__jki_lib_state_machine.vi"("State(s) in (\"\")"=w302) -> ("States Out"=w301:string)  [unwired: 14 in]
              }
              frame "Logger: Read Logger" {
                n102 = Unbundle By Name(w303) -> ()  [unwired: 1 out]
                n103 = call <vilib>:"Add State(s) to Queue__jki_lib_state_machine.vi"("State(s) in (\"\")"=w307) -> ("States Out"=w306:string)  [unwired: 14 in]
              }
              frame "Logger: Destroy Logger" {
                n104 = Unbundle By Name(w311) -> ("Self Reference"=w310:refnum<class "Logger.lvclass">)
                n105 = disable-structure shown="Enabled" {
                  disable-tunnel: w310 -> [w317 _]
                  disable-tunnel: w309 -> [w316 w318]
                  disable-tunnel: [w315 w318] -> w308
                  frame Disabled {
                    n106 = call-dynamic "Destroy Logger.vi"("error in (no error)"=w316, "Logger in"=w317) -> ("error out"=w315:errorcluster)  [unwired: 8 in, 1 out]
                  }
                  frame Enabled {
                  }
                }
                n107 = call <vilib>:"Add State(s) to Queue__jki_lib_state_machine.vi"("State(s) in (\"\")"=w314) -> ("States Out"=w313:string)  [unwired: 14 in]
              }
            }
          }
        }
        frame Error {
        }
      }
      n108 = call-parent "Process_DoNotRun.vi"("error in"=w9, "SMO"=w8) -> ("error out"=w6:errorcluster, "SMO out"=w7:refnum<class "Logger.lvclass">)  [unwired: 8 in]
      n109 = Merge Errors(w6, w5) -> (w10:errorcluster)
    }
    frame Enabled {
    }
  }
  "Logger out" <- w1
  "error out" <- w2
